vi "PPSU Detection 2.vi"(8 "error in":errorcluster, 10 "PPSU Dect 2":T1, 11 "Write/Read":enum16{"Write", "Read"}(ring)=enum."Read") -> (0 "error out":errorcluster, 2 "PPSU Dect":T1)   [LabVIEW 2022 SP3]
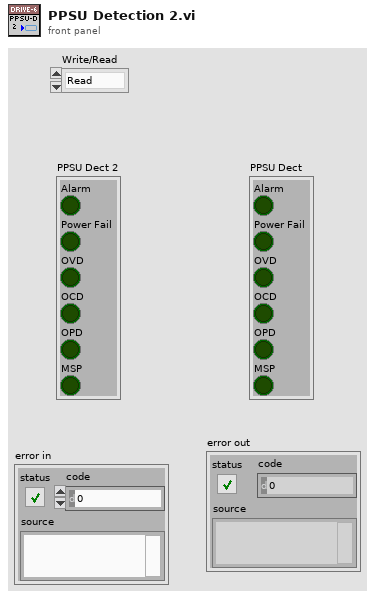
[diagram p1: front panel]
types:
  T1 = cluster{"Alarm":bool, "Power Fail":bool, "OVD":bool, "OCD":bool, "OPD":bool, "MSP":bool}
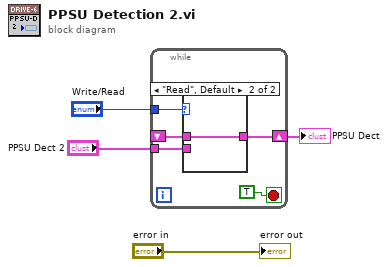
[diagram p0: block diagram]
diagram:
  n1 = while {
    tunnel: "Write/Read" -> [w9]
    tunnel: "PPSU Dect 2" -> [w7]
    shift-right: [w6] -> w1
    shift-left: _ -> [w5]
    stop <- TRUE stop-if-true
    n2 = case shown="\"Read\", Default" w9 {
      tunnel: w7 -> [w10 _]
      tunnel: [w10 w11] -> w6
      tunnel: w5 -> [_ w11]
      frame "Write" {
      }
      frame "Read", Default {
      }
    }
  }
  "PPSU Dect" <- w1
  "error out" <- "error in"
